vi "Create 1D Table.vi"(4 "use apostrophes (F)":bool, 5 "collumn vector (F)":bool, 8 "formatted values":string[](array[string]), 11 "table name":string) -> (0 "can be indented?":bool, 3 "table":string)   [LabVIEW 2019, in "infolib.lvlib"]
uses:
  infolib.lvlib
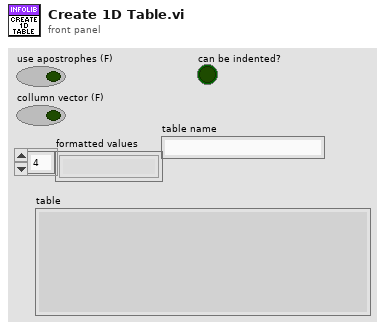
[diagram p1: front panel]
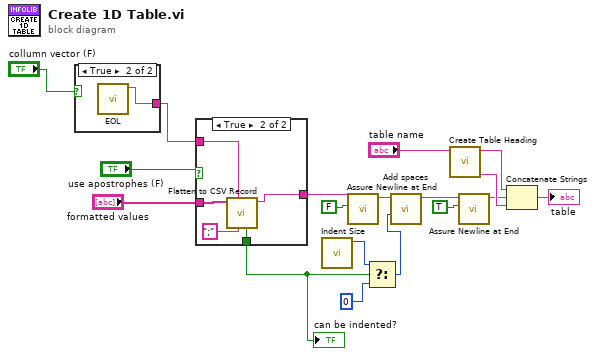
[diagram p0: block diagram]
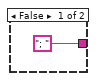
[diagram p2: hidden frame]
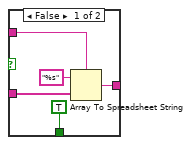
[diagram p3: hidden frame]
diagram:
  n1 = case shown="True" "collumn vector (F)" {
    tunnel: ["; " ("delimiter (Tab)") w20] -> w6
    frame False {
    }
    frame True {
      n2 = call "EOL.vi"() -> ("eol"=w20:string)  [unwired: 11 in]
    }
  }
  n3 = case shown="True" "use apostrophes (F)" {
    tunnel: "formatted values" -> [w25 w30]
    tunnel: [w24 w28] -> w8
    tunnel: w6 -> [w22 w29]
    tunnel: [TRUE ("can be indented?") w27] -> w2
    frame False {
      n4 = Array To Spreadsheet String(delimiter (Tab)=w22, array=w25, 3:"%s" ("format string")) -> (spreadsheet string=w24:string)
    }
    frame True {
      n5 = call "Flatten to CSV Record.vi"("regular expression - protected characters ([])"=";", "delimiter (,)"=w29, "row of strings"=w30) -> ("CSV record"=w28:string, "can be indented?"=w27:bool)  [unwired: 6 in, 1 out]
    }
  }
  "can be indented?" <- w2
  n6 = call "Indent Size.vi"() -> ("indent size"=w5:i32)  [unwired: 10 in, 1 out]
  n7 = call "Assure Newline at End.vi"("Set End Of Line (F)"=FALSE, "string"=w8) -> ("string out"=w14:string)  [unwired: 9 in]
  n8 = Select(t=w5, s=w2, f=0) -> (s? t:f=w4:i32)
  n9 = call "Add spaces.vi"("spaces no"=w4, "input string"=w14) -> ("result string"=w12:string)  [unwired: 9 in]
  n10 = call "Create Table Heading.vi"("table name"="table name") -> ("table end"=w16:string, "table start"=w17:string)  [unwired: 9 in]
  n11 = call "Assure Newline at End.vi"("Set End Of Line (F)"=TRUE, "string"=w12) -> ("string out"=w11:string)  [unwired: 9 in]
  n12 = Concatenate Strings(w17, w11, w16) -> (→"table":string)
